vi "Get uService Log Path.vi"(8 "error in (no error)":errorcluster, 10 "Log File Suffix":string, 11 "Father of all uServices in":refnum<class "Father of all uServices.lvclass">) -> (0 "error out":errorcluster, 2 "Log File Path":path, 3 "Father of all uServices out":refnum<class "Father of all uServices.lvclass">)   [LabVIEW 2026, in "TALOS.lvlib" / "Father of all uServices.lvlib" / "Father of all uServices.lvclass"]
doc: "VI for creating a dedicated directory for uS related logs. The directory path structure is <TALOS Log Path>/<uService ID>/<uService ID><suffix>"
uses:
  Father of all uServices.lvclass
  C:/LabVIEW Code/TALOS/talos/Ancestor/Ancestor/Ancestor.lvclass
  Ancestor/Ancestor/Ancestor.lvclass/Ancestor.ctl
  Ancestor/Ancestor/Read ID.vi
  Support VIs/Generate Error.vi
  FGV/Error Memory/Get Error Description.vi
  Support VIs/Get PC name.vi
  Support VIs/Get Class Name.vi
  <vilib>/Utility/error.llb/Clear Errors.vi
  FGV/Error Memory/Error Memory Core.vi
  <vilib>/AdvancedString/Delimited String to 1D String Array.vi
  <vilib>/AdvancedString/Delimited String to 1D String Array (string).vi
  Support VIs/Circus Root Path.vi
  FGV/Error Memory/Error Crt Lvl checker.vi
  FGV/Error Memory/Error Memory Core.vi/40c8088d-b597-4017-91af-faa98e00292e.vi
  FGV/Error Memory/Error Memory Core.vi/d4a3ab98-063c-4e44-b43d-fbdcfe6c2be2.vi
  Support VIs/Global Memory.vi
  <vilib>/Utility/LVClass/Get LV Class Name.vi
  Support VIs/Is in Packed Library.vi
  Support VIs/TALOS Root path.vi
  Support VIs/Read CSV worksheet.vi
  Support VIs/Global Constants.vi
  <vilib>/Utility/error.llb/General Error Handler.vi
  <vilib>/Utility/config.llb/Open Config Data.vi
  <vilib>/Utility/config.llb/Get Section Names.vi
  <vilib>/Utility/config.llb/Get Key Names.vi
  <vilib>/Utility/config.llb/Read Key.vi
  <vilib>/Utility/config.llb/Read Key (String).vi
  <vilib>/Utility/config.llb/Close Config Data.vi
  Support VIs/Error Log.vi
  Ancestor/Ancestor/Ancestor.lvclass
  <vilib>/Comparison/Equal/Equal Functor/Equal Functor.lvclass
  TALOS.lvlib
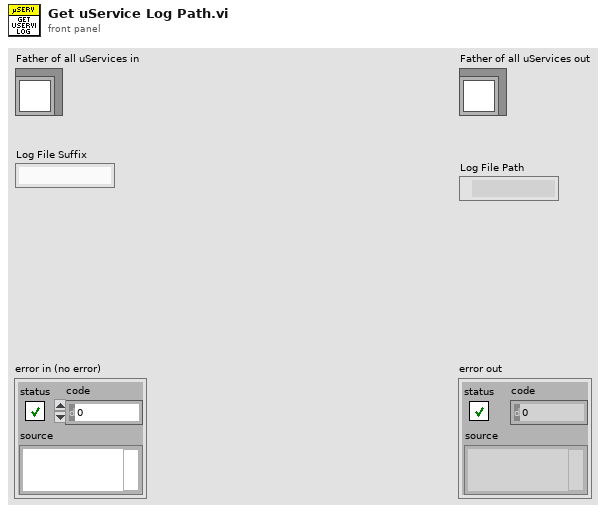
[diagram p1: front panel]
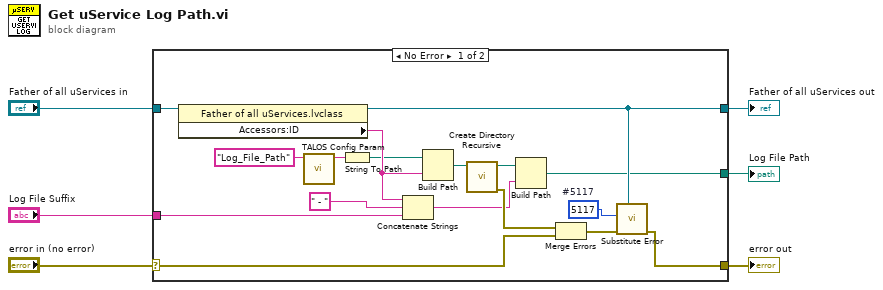
[diagram p0: block diagram]
diagram:
  n1 = case shown="No Error" "error in (no error)" {
    selector: "error in (no error)" -> [w13 w25]
    tunnel: [w10 w25] -> w5
    tunnel: [w9 w24] -> w3
    tunnel: "Father of all uServices in" -> [w22 w24]
    tunnel: "Log File Suffix" -> [w20 _]
    tunnel: [w8 _] -> w1
    frame No Error {
      w11 = 5117  # #5117
      n2 = property class="Father of all uServices.lvclass"(reference=w22) -> (reference out=w9:refnum<class "Father of all uServices.lvclass">, "Accessors:ID"=w21:string)  [unwired: 1 in, 1 out]
      n3 = call "TALOS Config Param.vi"("Parameter Name"="Log_File_Path") -> ("Output"=w18:string)  [unwired: 9 in, 1 out]
      n4 = String To Path(string=w18) -> (path=w17:path)
      n5 = Concatenate Strings(w21, " - " ("string"), w20) -> (w16:string)
      n6 = Build Path(base path=w17, name or relative path=w21) -> (appended path=w15:path)
      n7 = call <vilib>:"Create Directory Recursive.vi"("directory"=w15) -> ("error out"=w23:errorcluster, "directory copy"=w14:path)  [unwired: 4 in, 1 out]
      n8 = Build Path(base path=w14, name or relative path=w16) -> (appended path=w8:path)
      n9 = Merge Errors(w23, w13) -> (w12:errorcluster)
      n10 = call "Substitute Error.vi"("LabVIEW Object"=w9, "error in (no error)"=w12, "Error Code"=w11) -> ("error out"=w10:errorcluster)  [unwired: 8 in]
    }
    frame Error {
    }
  }
  "error out" <- w5
  "Father of all uServices out" <- w3
  "Log File Path" <- w1
